vi "版本判断.vi"() -> (3 "仪器类型":T1)   [LabVIEW 2016, in "斯坦道总磷.lvlib"]
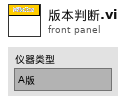
[diagram p1: front panel]
types:
  T1 = typedef "调试控件V3.xctl/仪器类型.ctl" = enum16{"A版", "B版"}
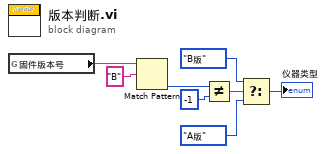
[diagram p0: block diagram]
diagram:
  n1 = global read "VAR总磷总氮全局变量.vi" "固件版本号"() -> (w1:string)
  n2 = Match Pattern(string=w1, regular expression="B" ("正则表达式")) -> (offset past match=w3:i32)  [unwired: 1 in, 3 out]
  n3 = Not Equal?(x=w3, y=-1) -> (x != y?=w5:bool)
  n4 = Select(t=仪器类型."B版" ("仪器类型"), s=w5, f=仪器类型."A版" ("仪器类型")) -> (s? t:f=→"仪器类型":T1)
